vi "Set Injected Value.vi"(8 "error in (no error)":errorcluster, 10 "Value":cdb, 11 "Fault-Insertion_Boolean_Type in":refnum<class "Fault-Injection_CDBL_Type.lvclass">) -> (0 "error out":errorcluster, 3 "Fault-Insertion_Boolean_Type out":refnum<class "Fault-Injection_CDBL_Type.lvclass">)   [LabVIEW 2021, in "Fault-Injection_CDBL_Type.lvclass"]
uses:
  Fault-Injection_CDBL_Type.lvclass
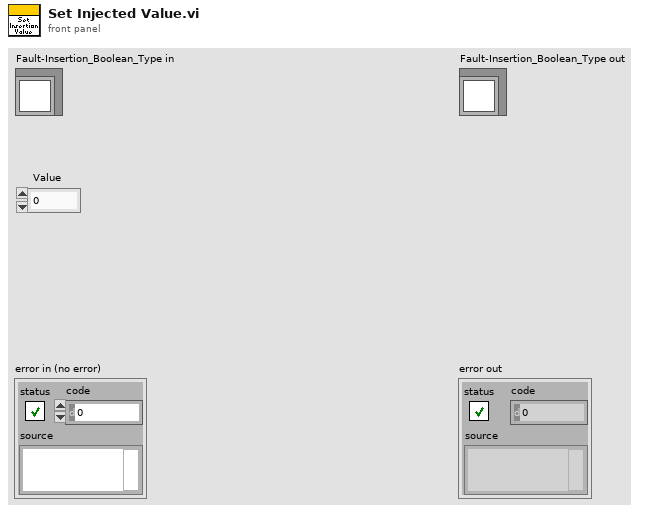
[diagram p1: front panel]
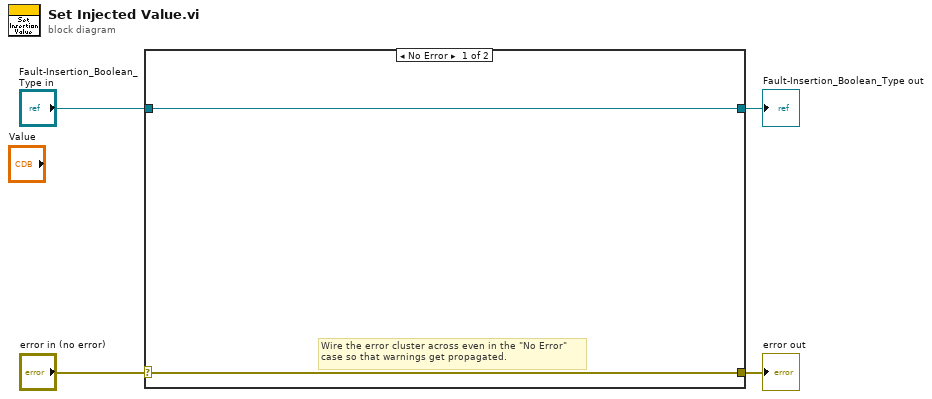
[diagram p0: block diagram]
diagram:
  n1 = case shown="No Error" "error in (no error)" {
    selector: "error in (no error)" -> [w5 w8]
    tunnel: [w5 w8] -> w3
    tunnel: [w6 w7] -> w1
    tunnel: "Fault-Insertion_Boolean_Type in" -> [w6 w7]
    frame No Error {
      # "Wire the error cluster across even in the \"No Error\"\ncase so that warnings get propagated."
    }
    frame Error {
    }
  }
  "error out" <- w3
  "Fault-Insertion_Boolean_Type out" <- w1
